vi "st_str Settings Dialog(VIForIzm).vi"(8 "error in (no error)":errorcluster, 11 "GenParametr":T1={"UgenVrms"=0.0, "Frequency 1,kHz"=0.0, "dFreq, kHz"=0.0, "Frequency 2,kHz"=0.0, "WaitSignalGen"=150.0}) -> (0 "error out":errorcluster, 2 "UI Refresh Needed?":bool, 3 "GenParametr":T1={"UgenVrms"=0.0, "Frequency 1,kHz"=0.0, "dFreq, kHz"=0.0, "Frequency 2,kHz"=0.0, "WaitSignalGen"=150.0})   [LabVIEW 2017]
doc: "Dialog for selecting user specified settings."
uses:
  controls/st_str gen parametr.ctl
  st_voltmetr/subVIs/st_str Global.vi
panel:
  in  "Задержка между шагом, mks(мин:1000)":dbl=1000.0
  in  "Frequency 2,kHz":dbl=270.0 caption="Конечная частота,kHz"
  in  "dFreq, kHz":dbl=10.0 caption="Шаг по частоте, kHz"
  in  "Frequency 1,kHz":dbl=10.0 caption="Начальная частота, kHz"
  in  "UgenVrms":dbl=1.0 caption="Напряжение. V"
  in  "Cancel Button":bool
  in  "OK Button":bool
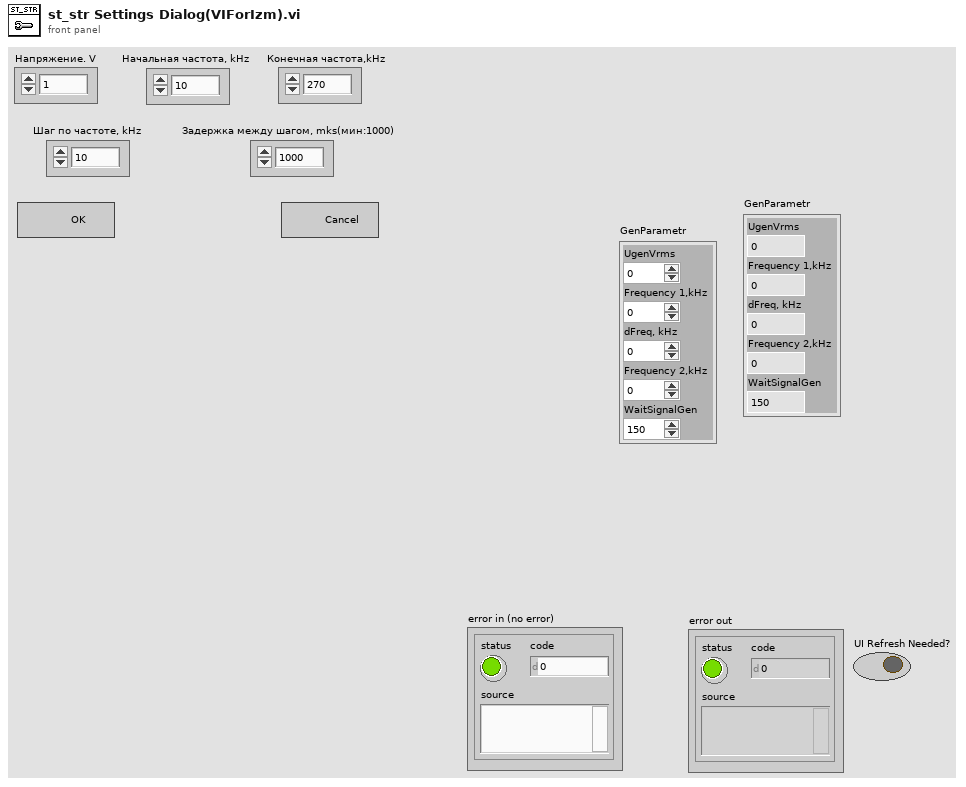
[diagram p1: front panel]
types:
  T1 = typedef "st_str gen parametr.ctl" = cluster{"UgenVrms":dbl, "Frequency 1,kHz":dbl, "dFreq, kHz":dbl, "Frequency 2,kHz":dbl, "WaitSignalGen":dbl}
  T2 = enum8{"Enabled", "Disabled", "Disabled and Grayed Out"}
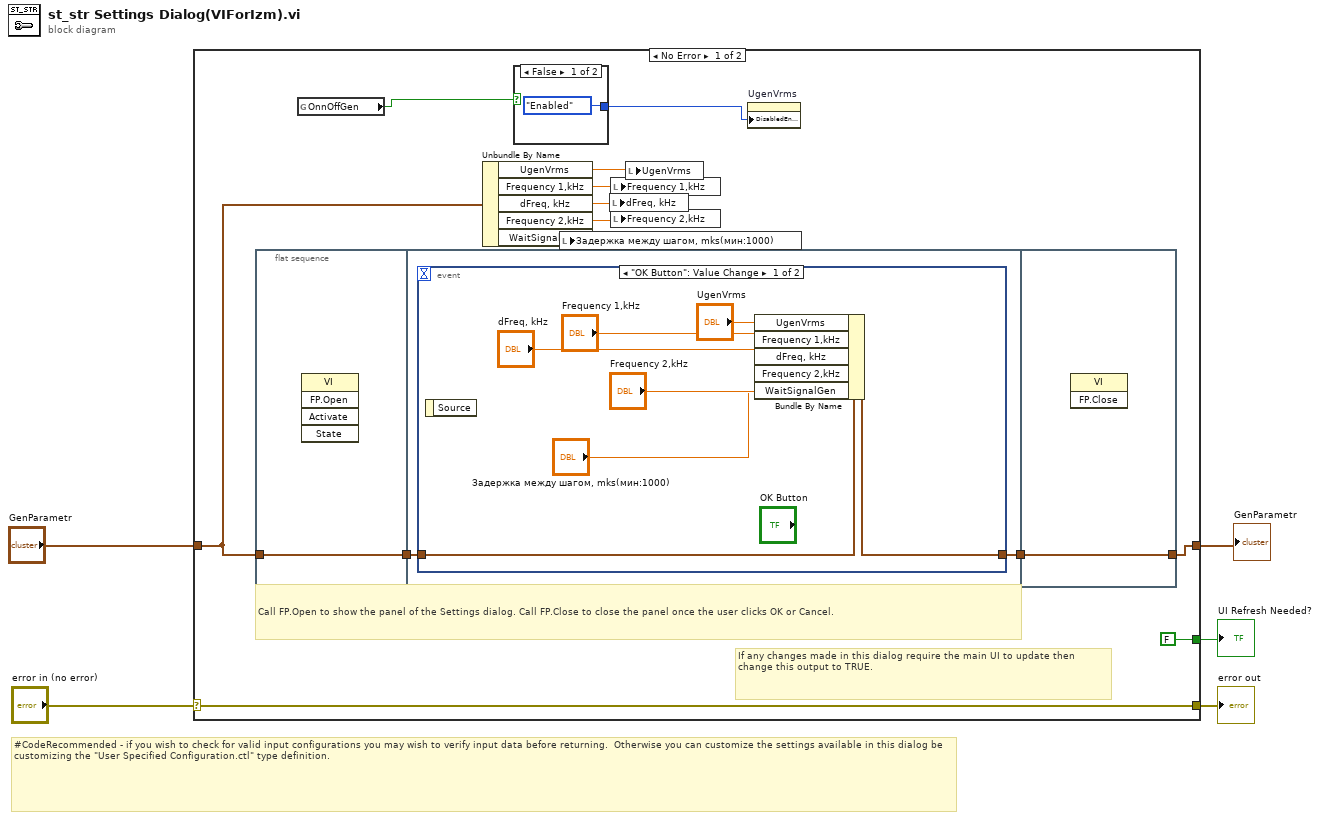
[diagram p0: block diagram]
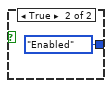
[diagram p2: hidden frame]
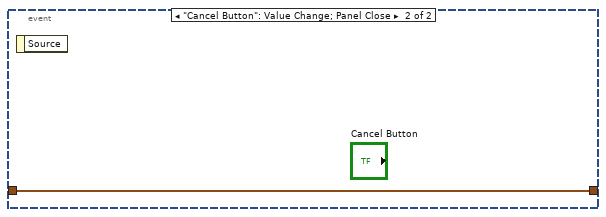
[diagram p3: hidden frame]
diagram:
  # "#CodeRecommended - if you wish to check for valid input configurations you may wish to verify input data before returning.  Otherwise you can customize the settings available in this dialog be customizing the \"User Specified Configuration.ctl\" type definition."
  n1 = case shown="No Error" "error in (no error)" {
    selector: "error in (no error)" -> [w18 w34]
    tunnel: [w18 w34] -> w4
    tunnel: "GenParametr" -> [w15 w33]
    tunnel: [w17 w33] -> w1
    tunnel: [FALSE ("UI Refresh Needed?") _] -> w2
    frame No Error {
      # "Call FP.Open to show the panel of the Settings dialog. Call FP.Close to close the panel once the user clicks OK or Cancel."
      # "If any changes made in this dialog require the main UI to update then change this output to TRUE."
      n2 = flat-sequence {
        tunnel: w15 -> [w21]
        tunnel: [w21] -> w14
        tunnel: w14 -> [w22]
        tunnel: [w23] -> w13
        tunnel: [w32] -> w17
        tunnel: w13 -> [w32]
        frame #0 {
          n3 = invoke class="VI" method="FP.Open"() -> ()  [unwired: 5 in, 5 out]
        }
        frame #1 {
          n4 = event shown="[0] \"OK Button\": Value Change" {
            selector: _ -> [_ _]
            dyn-events: _ -> [_ _]
            timeout: _ -> [_ _]
            tunnel: [w29 w31] -> w23
            tunnel: w22 -> [w30 w31]
            event "OK Button": Value Change {
              n5 = event-data() -> ()  [unwired: 1 in, 1 out]
              n6 = Bundle By Name(cluster=w30, "UgenVrms"="UgenVrms", "Frequency 1,kHz"="Frequency 1,kHz", "dFreq, kHz"="dFreq, kHz", "Frequency 2,kHz"="Frequency 2,kHz", "WaitSignalGen"="Задержка между шагом, mks(мин:1000)") -> (w29:T1)
            }
            event "Cancel Button": Value Change; Panel Close {
              n7 = event-data() -> ()  [unwired: 1 in, 1 out]
            }
          }
        }
        frame #2 {
          n8 = invoke class="VI" method="FP.Close"() -> ()  [unwired: 3 in, 3 out]
        }
      }
      n9 = global read "st_str Global.vi" "OnnOffGen"() -> (w7:bool)
      n10 = Unbundle By Name(w15) -> ("UgenVrms"=w12:dbl, "Frequency 1,kHz"=w11:dbl, "dFreq, kHz"=w10:dbl, "Frequency 2,kHz"=w9:dbl, "WaitSignalGen"=w8:dbl)
      n11 = case shown="False" w7 {
        tunnel: [T2."Enabled" ("Disabled") T2."Enabled" ("Disabled")] -> w6
        frame False {
        }
        frame True {
        }
      }
      n12 = local write "Задержка между шагом, mks(мин:1000)"(w8) -> ()
      n13 = local write "dFreq, kHz"(w10) -> ()
      n14 = local write "Frequency 1,kHz"(w11) -> ()
      n15 = local write "Frequency 2,kHz"(w9) -> ()
      n16 = local write "UgenVrms"(w12) -> ()
      n17 = property on="UgenVrms" class="DigNum (strict)"("DisabledEnum"=w6) -> ()  [unwired: 2 in, 2 out]
    }
    frame Error {
    }
  }
  "UI Refresh Needed?" <- w2
  "error out" <- w4
  "GenParametr" <- w1
